vi "Read SubPanel Event.vi"(11 "Base UI Component in":refnum<class "Base UI Component.lvclass">) -> (2 "SubPanel Event":refnum<user-event>)   [LabVIEW 2016, in "Assert API Components.lvlib" / "Assert Display.lvlib" / "Base UI Component.lvlib" / "Base UI Component.lvclass"]
uses:
  Base UI Component.lvclass
  Base UI Component.lvclass/Base UI Component.ctl
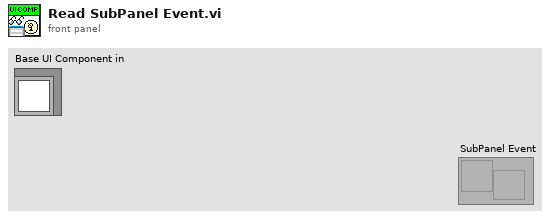
[diagram p1: front panel]
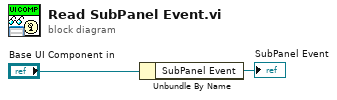
[diagram p0: block diagram]
diagram:
  n1 = Unbundle By Name("Base UI Component in") -> ("SubPanel Event"=→"SubPanel Event":refnum<user-event>)
